vi "Unpack (if allowable).vi"(11 "Observer in":refnum<class "Observer.lvclass">) -> (2 "Array out":refnum<class "Send.lvclass">[](array[class]))   [LabVIEW 2011, in "Messenging.lvlib" / "Observer.lvclass"]
uses:
  Observer.lvclass
  Send/Send.lvclass
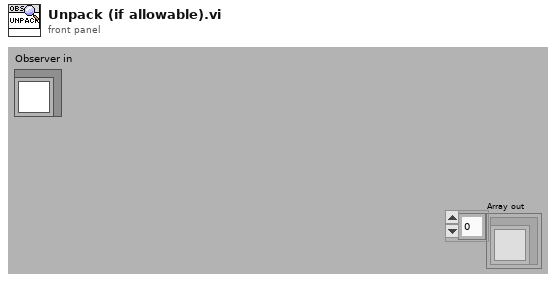
[diagram p1: front panel]
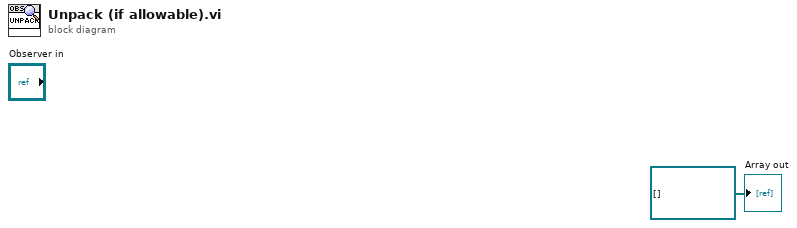
[diagram p0: block diagram]
diagram:
  "Array out" <- refnum<class "Send.lvclass">[] [] ("Array out")
